vi "AOTF_LaserChannel_6_FGV.vi"(8 "error in":errorcluster, 10 "Set_Get":u16(ring) items=["Set", "Get", "WaveformConvert"], 11 "LaserChannel_1_IN":T1) -> (0 "error out":errorcluster, 3 "LaserChannel_2_OUT":T1)   [LabVIEW 2011]
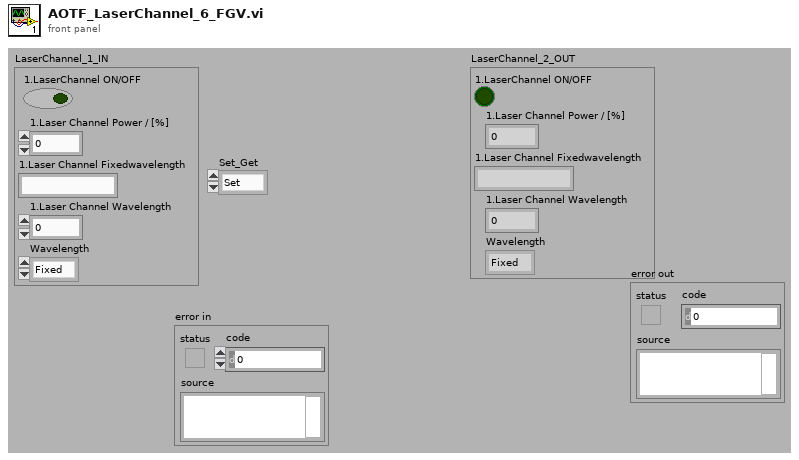
[diagram p1: front panel]
types:
  T1 = cluster{"1.LaserChannel ON/OFF":bool, "1.Laser Channel Power / [%]":i16, "1.Laser Channel Fixedwavelength":string, "1.Laser Channel Wavelength":i32, "Wavelength":enum16{"Fixed", "UserDefined"}}
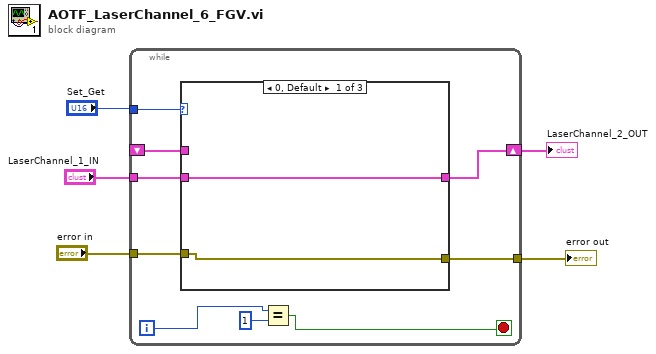
[diagram p0: block diagram]
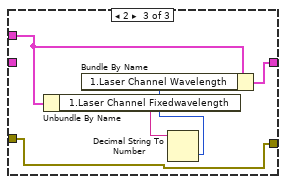
[diagram p3: hidden frame]
diagram:
  n1 = while {
    tunnel: "Set_Get" -> [w14]
    tunnel: "LaserChannel_1_IN" -> [w13]
    shift-right: [w12] -> w3
    shift-left: _ -> [w11]
    tunnel: [w7] -> w2
    tunnel: "error in" -> [w6]
    i -> [w8]
    stop <- w9 stop-if-true
    n2 = case shown="0, Default" w14 {
      tunnel: w13 -> [w16 _ _]
      tunnel: [w16 w17 w19] -> w12
      tunnel: w11 -> [_ w17 w20]
      tunnel: [w15 _ w18] -> w7
      tunnel: w6 -> [w15 _ w18]
      frame 0, Default {
      }
      frame 1 {
      }
      frame 2 {
        n3 = Unbundle By Name(w20) -> ("1.Laser Channel Fixedwavelength"=w22:string)
        n4 = Decimal String To Number(string=w22) -> (number=w21:i32)  [unwired: 2 in, 1 out]
        n5 = Bundle By Name(cluster=w20, "1.Laser Channel Wavelength"=w21) -> (w19:T1)
      }
    }
    n6 = Equal?(x=w8, y=1) -> (x = y?=w9:bool)
  }
  "LaserChannel_2_OUT" <- w3
  "error out" <- w2
